vi "SSC DCPower Get and Set Source Delay for Multiple Pins.vi"(0 "DCPower SSC in":T1[](array[typedef]), 7 "New Source Delay":dbl, 11 "error in":errorcluster) -> (4 "DCPower SSC out":T1[](array[typedef]), 8 "Current Source Delay":dbl[](array[numeric]), 15 "error out":errorcluster)   [LabVIEW 2019]
uses:
  SSC DCPower.ctl
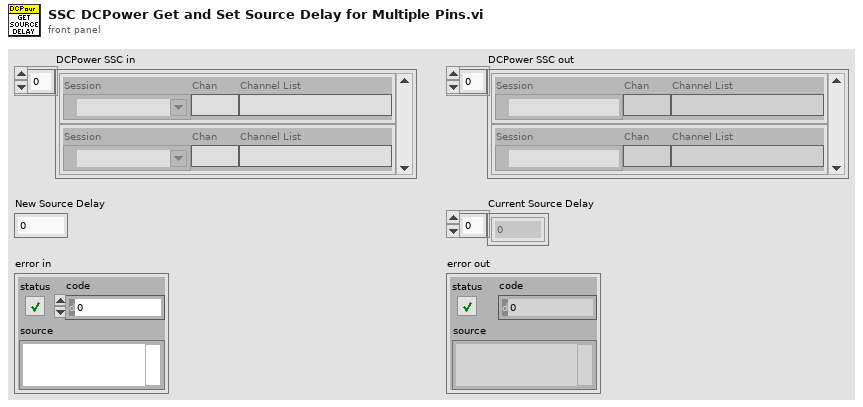
[diagram p1: front panel]
types:
  T1 = typedef "SSC DCPower.ctl" = cluster{"Session":refnum<k15>, "Chan":string, "Channel List":string}
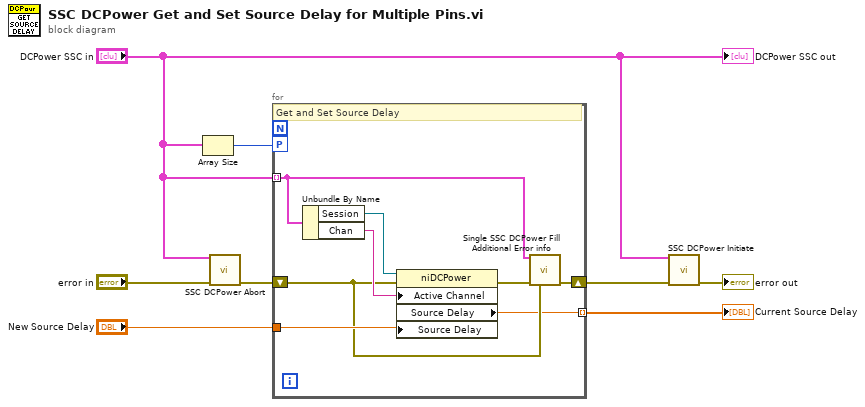
[diagram p0: block diagram]
diagram:
  n1 = Array Size(array="DCPower SSC in") -> (size(s)=w8:i32)
  n2 = call "SSC DCPower Abort.vi"("DCPower SSC in"="DCPower SSC in", "error in"="error in") -> ("error out"=w6:errorcluster)  [unwired: 12 in, 1 out]
  n3 = for {
    tunnel: "DCPower SSC in" -> [w13] mode=indexing
    workers-P: w8 -> [_]
    shift-right: [w11] -> w5
    shift-left: w6 -> [w10]
    tunnel: "New Source Delay" -> [w14]
    tunnel: [w9] -> w1 mode=indexing
    # "Get and Set Source Delay"
    n4 = Unbundle By Name(w13) -> ("Session"=w16:refnum<k15>, "Chan"=w15:string)
    n5 = property class="niDCPower"(reference=w16, error in=w10, "Active Channel"=w15, "Source Delay"=w14) -> (error out=w12:errorcluster, "Source Delay"=w9:dbl)  [unwired: 1 out]
    n6 = call "Single SSC DCPower Fill Additional Error info.vi"("DCPower SSC in"=w13, "error in"=w12, "previous error in"=w10) -> ("error out"=w11:errorcluster)  [unwired: 12 in]
  }
  "Current Source Delay" <- w1
  n7 = call "SSC DCPower Initiate.vi"("DCPower SSC in"="DCPower SSC in", "error in"=w5) -> ("error out"=→"error out":errorcluster)  [unwired: 12 in, 1 out]
  "DCPower SSC out" <- "DCPower SSC in"
